vi "Get Parameter Original Indices.vi"(11 "Parameter Types":bool[](array[boolean])) -> (0 "Global Fit Parameter Info":T1, 2 "Plot Specific Parameter Indices":i32[](array[numeric]), 3 "Global Parameter Indices":i32[](array[numeric]))   [LabVIEW 2021]
uses:
  Global Fit Parameters Information.ctl
  Fits.lvlib
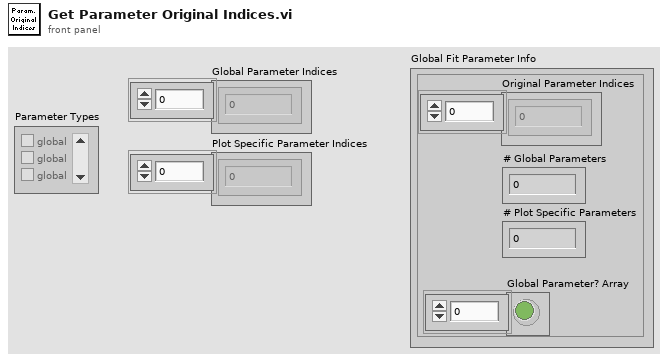
[diagram p1: front panel]
types:
  T1 = typedef "Fits.lvlib/Global Fit Parameters Information.ctl" = cluster{"Original Parameter Indices":i32[], "# Global Parameters":i32, "# Plot Specific Parameters":i32, "Global Parameter? Array":bool[]}
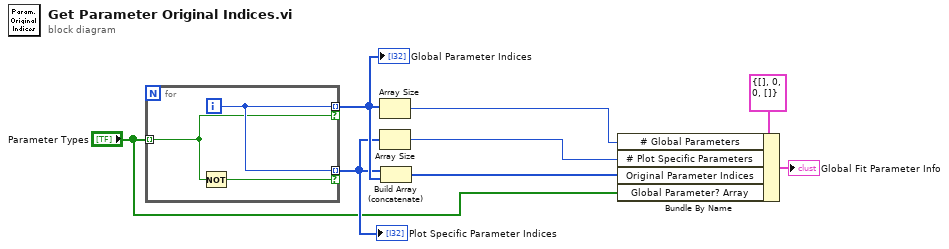
[diagram p0: block diagram]
diagram:
  n1 = for {
    tunnel: "Parameter Types" -> [w10] mode=indexing
    tunnel: [w11] -> w8 mode=indexing if=w10
    tunnel: [w11] -> w7 mode=indexing if=w9
    i -> [w11]
    n2 = Not(x=w10) -> (.not. x?=w9:bool)
  }
  "Global Parameter Indices" <- w8
  "Plot Specific Parameter Indices" <- w7
  n3 = Array Size(array=w8) -> (size(s)=w4:i32)
  n4 = Array Size(array=w7) -> (size(s)=w5:i32)
  n5 = Build Array (concatenate)(w7, w8) -> (w6:i32[])
  n6 = Bundle By Name(cluster=T1 {"Original Parameter Indices"=[], "# Global Parameters"=0, "# Plot Specific Parameters"=0, "Global Parameter? Array"=[]} ("Global Fit Parameter Info"), "# Global Parameters"=w4, "# Plot Specific Parameters"=w5, "Original Parameter Indices"=w6, "Global Parameter? Array"="Parameter Types") -> (→"Global Fit Parameter Info":T1)
